vi "mW_store_DATA.vi"(0 "file path (dialog if empty)":path, 1 "Eventnum":dbl, 2 "ADC":dbl, 3 "Posittion":dbl, 4 "Polarization":dbl, 5 "Frequency":dbl, 8 "error in (no error)":errorcluster) -> (14 "new file path (Not A Path if cancelled)":path, 19 "error out":errorcluster)   [LabVIEW 2019]
uses:
  <vilib>/Utility/file.llb/Write Delimited Spreadsheet (DBL).vi
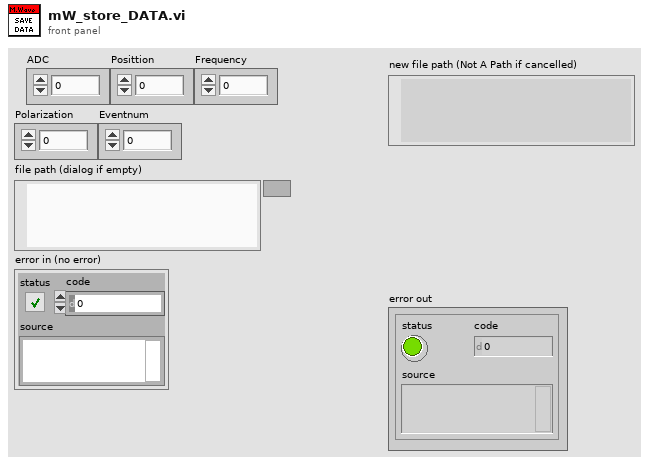
[diagram p1: front panel]
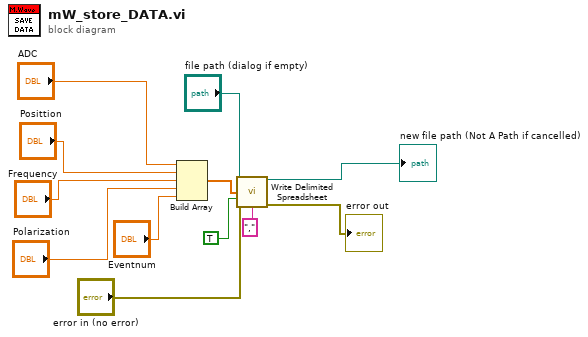
[diagram p0: block diagram]
diagram:
  n1 = Build Array("ADC", "Posittion", "Frequency", "Polarization", "Eventnum") -> (w10:dbl[])
  n2 = call-poly <vilib>:"Write Delimited Spreadsheet.vi"("file path (dialog if empty)"="file path (dialog if empty)", "1D data"=w10, "append to file? (new file:F)"=TRUE, "error in (no error)"="error in (no error)", "delimiter (\\t)"="," ("delimiter (\\t)")) -> ("new file path (Not A Path if cancelled)"=→"new file path (Not A Path if cancelled)":path, "error out"=→"error out":errorcluster)  [unwired: 9 in]
